vi "Local Dispatch Loop.vi"(8 "error in (no error)":errorcluster, 11 "TCPMessaging in":refnum<class "TCPMessaging.lvclass">) -> (0 "error out":errorcluster)   [LabVIEW 2020, in "Vecto.lvlib" / "TCPMessaging.lvclass"]
uses:
  TCPMessaging.lvclass
  TCPMessaging.lvclass/TCPMessaging.ctl
  TCPMessageHandler/TCPMessageHandler.lvclass
  proto/TcpPayload/TcpPayload.lvlib
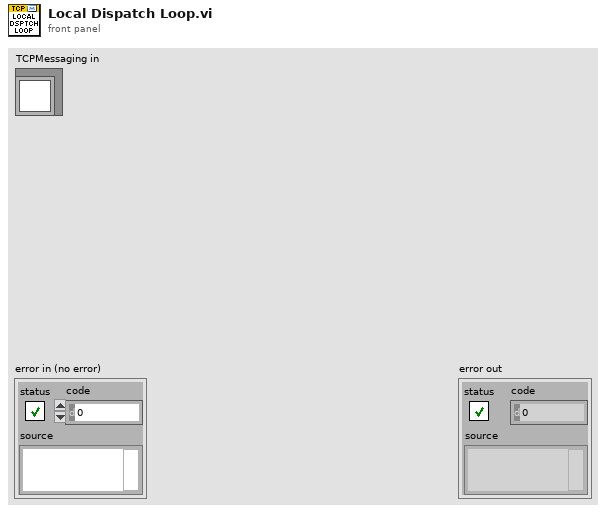
[diagram p1: front panel]
types:
  T1 = typedef "TcpPayload.lvlib/Data.ctl" = cluster{"target_node":u32, "target_task":u32, "source_id":u32, "sequence":u32, "timestamp":u64, "type_id":u32, "payload":u8[]}
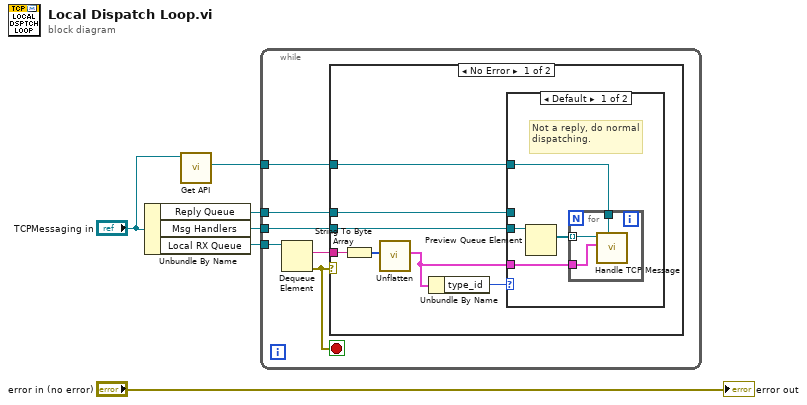
[diagram p0: block diagram]
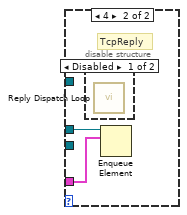
[diagram p2: hidden frame]
diagram:
  n1 = Unbundle By Name("TCPMessaging in") -> ("Reply Queue"=w1:refnum<queue>, "Msg Handlers"=w4:refnum<queue>, "Local RX Queue"=w5:refnum<queue>)
  n2 = call "Get API.vi"("TCPMessaging in"="TCPMessaging in") -> ("TCP Messaging API"=w2:refnum<class "TCPMessageAPI.lvclass">)  [unwired: 8 in, 2 out]
  n3 = while {
    tunnel: w5 -> [w12]
    tunnel: w4 -> [w11]
    tunnel: w2 -> [w9]
    tunnel: w1 -> [w7]
    stop <- w8 stop-if-true
    n4 = Dequeue Element(queue=w12) -> (element=w10:string, error out=w8:errorcluster)  [unwired: 2 in, 2 out]
    n5 = case shown="No Error" w8 {
      tunnel: w11 -> [w19 _]
      tunnel: w10 -> [w18 _]
      tunnel: w9 -> [w16 _]
      tunnel: w7 -> [w13 _]
      frame No Error {
        n6 = String To Byte Array(string=w18) -> (unsigned byte array=w17:u8[])
        n7 = call "Unflatten.vi"("Buffer"=w17) -> ("Data"=w15:T1)  [unwired: 9 in, 1 out]
        n8 = Unbundle By Name(w15) -> ("type_id"=w14:u32)
        n9 = case shown="Default" w14 {
          tunnel: w19 -> [w23 _]
          tunnel: w16 -> [w21 _]
          tunnel: w15 -> [w20 w27]
          tunnel: w13 -> [_ w28]
          frame Default {
            # "Not a reply, do normal dispatching."
            n10 = Preview Queue Element(queue=w23) -> (element=w22:refnum<class "TCPMessageHandler.lvclass">[])  [unwired: 2 in, 3 out]
            n11 = for {
              tunnel: w22 -> [w26] mode=indexing
              tunnel: w21 -> [w25]
              tunnel: w20 -> [w24]
              n12 = call-dynamic "Handle TCP Message.vi"("TCPMessageAPI"=w25, "TcpPayload"=w24, "TCPMessageHandler in"=w26) -> ()  [unwired: 7 in, 2 out]
            }
          }
          frame 4 {
            # "TcpReply"
            n13 = disable-structure shown="Disabled" {
              frame Disabled {
                n14 = call "Reply Dispatch Loop.vi"() -> ()  [unwired: 11 in, 1 out]
              }
              frame Enabled {
              }
            }
            n15 = Enqueue Element(queue=w28, element=w27) -> ()  [unwired: 2 in, 3 out]
          }
        }
      }
      frame Error {
      }
    }
  }
  "error out" <- "error in (no error)"
